vi "Publish AI.vi"(8 "error in":errorcluster, 10 "AI Data":dbl[](array[numeric]), 11 "BNT_DAQmx-MCSV in":refnum<class "BNT_DAQmx-MCSV.lvclass">) -> (0 "error out":errorcluster, 3 "BNT_DAQmx-MCSV out":refnum<class "BNT_DAQmx-MCSV.lvclass">)   [LabVIEW 2021, in "BNT_DAQmx.lvlib" / "BNT_DAQmx-MCSV.lvclass"]
doc: "Publish analog input values if greater than uncertainty."
uses:
  BNT_DAQmx-MCSV.lvclass
  BNT_DAQmx-MCSV.lvclass/BNT_DAQmx-MCSV.ctl
  CSPP_Core/Classes/CSPP_ProcessVariables/PVConnection/PVConnection.lvclass/PVConnection.ctl
  CSPP_Core/Classes/CSPP_ProcessVariables/ProcessVariable/PV.lvclass/PV.ctl
  CSPP_Core/Classes/CSPP_ProcessVariables/ProcessVariable/Write Data.vi
  CSPP_Core/Classes/CSPP_ProcessVariables/ProcessVariable/Write Error.vi
  CSPP_Core/Classes/CSPP_ProcessVariables/ProcessVariable/Write Quality.vi
  CSPP_Core/Classes/CSPP_ProcessVariables/ProcessVariable/Write status.vi
  CSPP_Core/Classes/CSPP_ProcessVariables/ProcessVariable/Write Timestamp.vi
  CSPP_Core/Classes/CSPP_ProcessVariables/ProcessVariable/PV.lvclass
  CSPP_Core/Classes/CSPP_ProcessVariables/PVConnection/PVConnection.lvclass
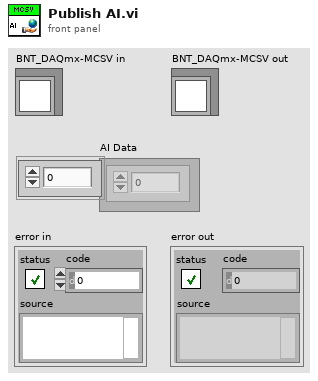
[diagram p1: front panel]
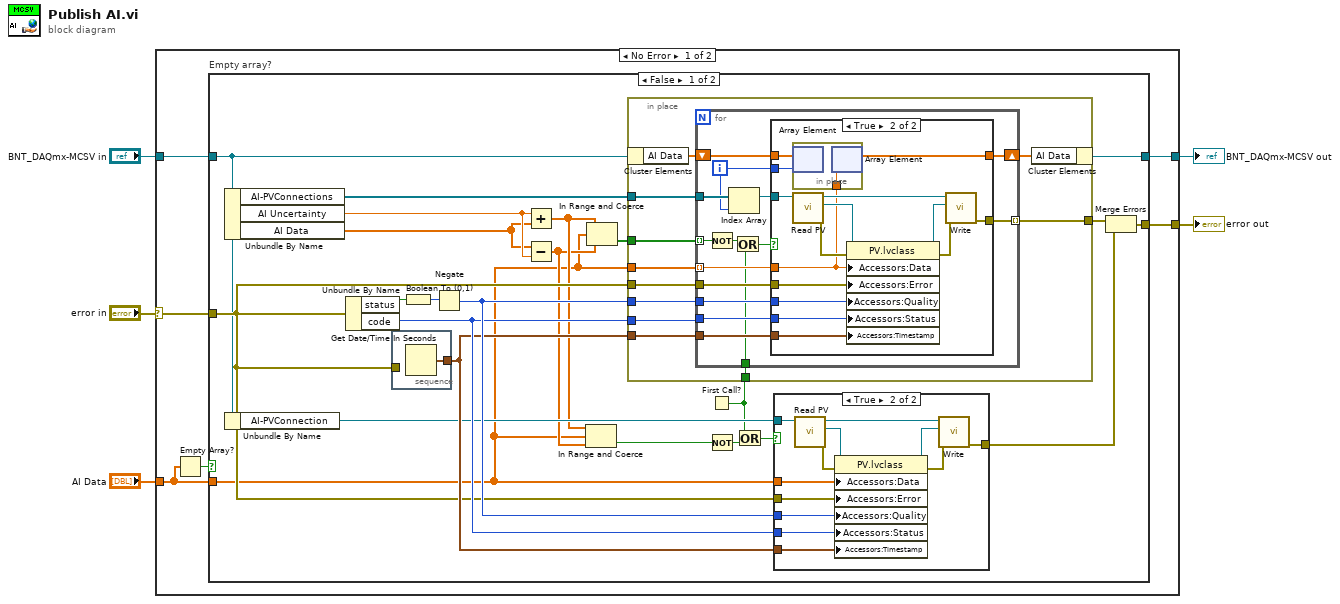
[diagram p0: block diagram]
diagram:
  n1 = case shown="No Error" "error in" {
    selector: "error in" -> [w11 w96]
    tunnel: [w10 w96] -> w4
    tunnel: [w8 w95] -> w2
    tunnel: "BNT_DAQmx-MCSV in" -> [w9 w95]
    tunnel: "AI Data" -> [w6 _]
    frame No Error {
      n2 = Empty Array?(array=w6) -> (empty?=w7:bool)
      n3 = case "Empty array?" shown="False" w7 {
        tunnel: w11 -> [w27 w93]
        tunnel: [w25 w93] -> w10
        tunnel: w6 -> [w14 _]
        tunnel: w9 -> [w18 w94]
        tunnel: [w17 w94] -> w8
        frame False {
          n4 = Unbundle By Name(w18) -> ("AI-PVConnections"=w26:refnum<class "PVConnection.lvclass">[], "AI Uncertainty"=w23:dbl, "AI Data"=w21:dbl[])
          n5 = Unbundle By Name(w18) -> ("AI-PVConnection"=w24:refnum<class "PVConnection.lvclass">)
          n6 = Unbundle By Name(w27) -> ("status"=w33:bool, "code"=w30:i32)
          n7 = stacked-sequence {
            tunnel: [w79] -> w29
            tunnel: w27 -> [_]
            frame #0 {
              n8 = Get Date/Time In Seconds() -> (seconds since 1Jan1904=w79:timestamp)
            }
          }
          n9 = Boolean To (0,1)(Boolean=w33) -> (0, 1=w32:i16)
          n10 = Negate(x=w32) -> (-x=w31:i16)
          n11 = Add(x=w23, y=w21) -> (x+y=w20:dbl[])
          n12 = Subtract(x=w21, y=w23) -> (x-y=w19:dbl[])
          n13 = In Range and Coerce(upper limit=w20, x=w14, lower limit=w19) -> (In Range?=w16:bool)  [unwired: 1 out]
          n14 = In Range and Coerce(upper limit=w20, x=w14, lower limit=w19) -> (In Range?=w22:bool[])  [unwired: 1 out]
          n15 = First Call?() -> (First Call?: T/F=w13:bool)
          n16 = in-place {
            in-place-border: [w45] -> w34
            in-place-border: w31 -> [w44]
            in-place-border: w30 -> [w43]
            in-place-border: w29 -> [w42]
            in-place-border: w27 -> [w41]
            in-place-border: w26 -> [w40]
            in-place-border: w14 -> [w39]
            in-place-border: w22 -> [w38]
            in-place-border: w13 -> [w35]
            n17 = in-place-cluster #1(w18) -> ("AI Data"=w37:dbl[])
            n18 = for {
              tunnel: w40 -> [w54]
              tunnel: w39 -> [w60] mode=indexing
              tunnel: w41 -> [w59]
              tunnel: [w58] -> w45 mode=indexing
              tunnel: w44 -> [w57]
              tunnel: w43 -> [w56]
              tunnel: w42 -> [w55]
              tunnel: w38 -> [w53] mode=indexing
              shift-right: [w51] -> w36
              shift-left: w37 -> [w52]
              tunnel: w35 -> [w49]
              i -> [w46]
              n19 = Not(x=w53) -> (.not. x?=w48:bool)
              n20 = Index Array(array=w54, index=w46) -> (element=w47:refnum<class "PVConnection.lvclass">)
              n21 = Or(x=w48, y=w49) -> (x .or. y?=w50:bool)
              n22 = case shown="True" w50 {
                tunnel: w60 -> [_ w64]
                tunnel: w59 -> [w62 w77]
                tunnel: [w62 w74] -> w58
                tunnel: w57 -> [_ w73]
                tunnel: w56 -> [_ w72]
                tunnel: w55 -> [_ w71]
                tunnel: w47 -> [_ w70]
                tunnel: w46 -> [_ w66]
                tunnel: w52 -> [w61 w65]
                tunnel: [w61 w63] -> w51
                frame False {
                }
                frame True {
                  n23 = in-place {
                    in-place-border: w64 -> [w78]
                    n24 = in-place-array #2(w65, w66) -> ()  [unwired: 1 out]
                    n25 = in-place-array #2(w78) -> (w63:dbl[])  [unwired: 1 out]
                  }
                  n26 = call "Read PV.vi"("PVConnection in"=w70) -> ("error out"=w67:errorcluster, "PV"=w68:refnum<class "PV.lvclass">, "PVConnection out"=w69:refnum<class "PVConnection.lvclass">)  [unwired: 8 in]
                  n27 = property class="PV.lvclass"(reference=w68, error in=w67, "Accessors:Data"=w64, "Accessors:Error"=w77, "Accessors:Quality"=w73, "Accessors:Status"=w72, "Accessors:Timestamp"=w71) -> (reference out=w76:refnum<class "PV.lvclass">, error out=w75:errorcluster)
                  n28 = call "Write.vi"("error in (no error)"=w75, "PV"=w76, "PVConnection in"=w69) -> ("error out"=w74:errorcluster)  [unwired: 6 in, 2 out]
                }
              }
            }
            n29 = in-place-cluster #1("AI Data"=w36) -> (w17:refnum<class "BNT_DAQmx-MCSV.lvclass">)
          }
          n30 = Not(x=w16) -> (.not. x?=w12:bool)
          n31 = Or(x=w13, y=w12) -> (x .or. y?=w15:bool)
          n32 = case shown="True" w15 {
            tunnel: w31 -> [_ w87]
            tunnel: w30 -> [_ w86]
            tunnel: w29 -> [_ w85]
            tunnel: [w80 w84] -> w28
            tunnel: w27 -> [w80 w83]
            tunnel: w24 -> [_ w82]
            tunnel: w14 -> [_ w81]
            frame False {
            }
            frame True {
              n33 = call "Read PV.vi"("PVConnection in"=w82) -> ("error out"=w88:errorcluster, "PV"=w89:refnum<class "PV.lvclass">, "PVConnection out"=w90:refnum<class "PVConnection.lvclass">)  [unwired: 8 in]
              n34 = property class="PV.lvclass"(reference=w89, error in=w88, "Accessors:Data"=w81, "Accessors:Error"=w83, "Accessors:Quality"=w87, "Accessors:Status"=w86, "Accessors:Timestamp"=w85) -> (reference out=w92:refnum<class "PV.lvclass">, error out=w91:errorcluster)
              n35 = call "Write.vi"("error in (no error)"=w91, "PV"=w92, "PVConnection in"=w90) -> ("error out"=w84:errorcluster)  [unwired: 6 in, 2 out]
            }
          }
          n36 = Merge Errors(w34, w28) -> (w25:errorcluster)
        }
        frame True {
        }
      }
    }
    frame Error {
    }
  }
  "error out" <- w4
  "BNT_DAQmx-MCSV out" <- w2
